vi "MotorControlMina4 with Joystick control2.vi"() -> ()   [LabVIEW 2014]
uses:
  <vilib>/Utility/inputDevices.llb/joystickAcquire.vi
  <vilib>/Utility/inputDevices.llb/closeJoystick.vi
panel:
  out "joystick info":T1(array[cluster])
  in  "Stop":bool
  out "InstrumentMode":T2(ring)=enum."Shutdown"
  in  "XMotorRef":refnum<k7>(container)
  in  "YMotorRef":refnum<k7>(container)
  in  "ZMotorRef":refnum<k7>(container)
  out "JoystOffset":T3={"XOffset"=-99999, "YOffset"=-99999, "ZOffset"=-99999}
  out "RelJoyPos":T4
  in  "InterfaceSelector":T5(tab)
  in  "GoToTopDisp":bool
  in  "GoToBottDisp":bool
  in  "GoToExpLoc":bool
  in  "SaveTopDisp":bool
  in  "SaveBottDisp":bool
  in  "SaveExpLoc":bool
  out "Top Dispenser":T6={"X Pos (mm)"=0.5532008, "Y Pos (mm)"=0.030929338, "Z Pos (mm)"=0.77973413} {"Y Pos (mm)" format="%.3f"; "Z Pos (mm)" format="%.3f"; "X Pos (mm)" format="%.3f"}
  out "Bottom Dispenser":T6={"X Pos (mm)"=0.600309, "Y Pos (mm)"=-1.1540928, "Z Pos (mm)"=0.7938141} {"Y Pos (mm)" format="%.3f"; "Z Pos (mm)" format="%.3f"; "X Pos (mm)" format="%.3f"}
  out "Experiment Region":T6={"X Pos (mm)"=1.4278219, "Y Pos (mm)"=-0.74810517, "Z Pos (mm)"=0.7938141} {"Y Pos (mm)" format="%.3f"; "Z Pos (mm)" format="%.3f"; "X Pos (mm)" format="%.3f"}
  in  "PreviewPanel":T7(tab)
  in  "Z Motor Settings":T8={"Joyst Min Signal"=10.0, "Joyst Max Signal"=30000.0, "Vmax (mm/s)"=0.005, "Acc (mm/s/s)"=0.2, "+ JoystDirection"=2, "- JoystDirection"=1} {"Acc (mm/s/s)" format="%#.3f"; "Vmax (mm/s)" format="%#.3f"}
  in  "Y Motor Settings":T8={"Joyst Min Signal"=10.0, "Joyst Max Signal"=20000.0, "Vmax (mm/s)"=0.03, "Acc (mm/s/s)"=0.5, "+ JoystDirection"=1, "- JoystDirection"=2} {"Acc (mm/s/s)" format="%#.3f"; "Vmax (mm/s)" format="%#.3f"}
  in  "X Motor Settings":T8={"Joyst Min Signal"=10.0, "Joyst Max Signal"=20000.0, "Vmax (mm/s)"=0.03, "Acc (mm/s/s)"=0.5, "+ JoystDirection"=2, "- JoystDirection"=1} {"Acc (mm/s/s)" format="%#.3f"; "Vmax (mm/s)" format="%#.3f"}
  in  "Motor Cruise Param":T9={"X Acc (mm/s^2)"=0.3, "X Vmax (mm/s)"=0.3, "Y Acc (mm/s^2)"=0.3, "Y Vmax (mm/s)"=0.3, "Z Acc (mm/s^2)"=0.1, "Z Vmax (mm/s)"=0.1}
  in  "Motor Limits":T10={"XMin"=-0.8, "XMax"=3.0, "YMin"=-2.0, "YMax"=2.0, "ZMin"=0.0, "ZMax"=2.0}
  in  "Steerable Mirror Calibration":T11={"Hor. Scaling (nm/V)"=760.0, "Vert. Scaling (nm/V)"=760.0, "Hor. Mirr. Offset (V)"=0.0, "Vert. Mirr. Offset (V)"=0.0}
  in  "Steerable \nTrap\n(F12)":bool
  in  "Fixed\nTrap\n(F11)":bool
  in  "Align Traps Vertically":bool
  in  "MaxHorizontalTrapSeparation":bool
  out "X Motor State":T12={"Direction"=0, "Vel (mm/s)"=0.0, "IsActive?"=FALSE, "Pos (mm)"=-0.2957381} {"Pos (mm)" format="%#.3f"; "Vel (mm/s)" format="%#.4f"}
  out "Y Motor State":T12={"Direction"=0, "Vel (mm/s)"=0.0, "IsActive?"=FALSE, "Pos (mm)"=0.016441232} {"Pos (mm)" format="%#.3f"; "Vel (mm/s)" format="%#.4f"}
  out "Z Motor State":T12={"Direction"=0, "Vel (mm/s)"=0.0, "IsActive?"=FALSE, "Pos (mm)"=-0.26253498} {"Pos (mm)" format="%#.3f"; "Vel (mm/s)" format="%#.4f"}
  out "Move Z":bool
  out "Move XY":bool
  in  "MotorLoopDelay":u32=100
  in  "StopPassiveMode":bool caption="stop"
  in  "PMVertSlider(V)":dbl(slide)=0.005145263671875 scale=0.0..10.0 scale format="%#_3f"
  in  "PMHorizSlider(V)":dbl(slide)=0.0045623779296875 scale=2.0..10.0
  out "IsPassiveModeActive?":bool caption="stop"
  out "Force TrapA":cluster{"x":dbl[], "y":dbl[]}[](graph)
  out "Noise-Ext":cluster{"x":dbl[], "y":dbl[]}[](graph)
  out "Force TrapB":cluster{"x":dbl[], "y":dbl[]}[](graph)
  out "IsOffsetModeActive?":bool caption="stop"
  in  "StopOffset":bool caption="stop"
  out "IsForceExtActive?":bool=TRUE
  in  "StopForceExtension":bool caption="stop"
  # "ClpXP Optical Tweezers"
  # "Chamber Locations"
  # "Need a Button Here that would read the \nNormalized Offset and save it"
  # "Off"
  # "On"
  # "Off"
  # "On"
  # "Thorlabs Motor Status"
  # "Passive Mode"
  # "when I switch tabs from the passive mode to basic mode, the recording doesn't stop"
  # "The sliders don't do anything in passive mode, fix it"
  # "Whenever I click on Ackquire Offset, it goes back to the basic operation, then I have to ckick again"
  # "Trap Motion Control"
  # "Steerable Mirror Info"
  # "Zero-Force Offset Mode"
  # "High Frequency Data Acquisition"
  # "Adjust the length of acquisition time"
  # "Force-Extension Mode"
  # "Y"
  # "+"
  # "X"
  # "-"
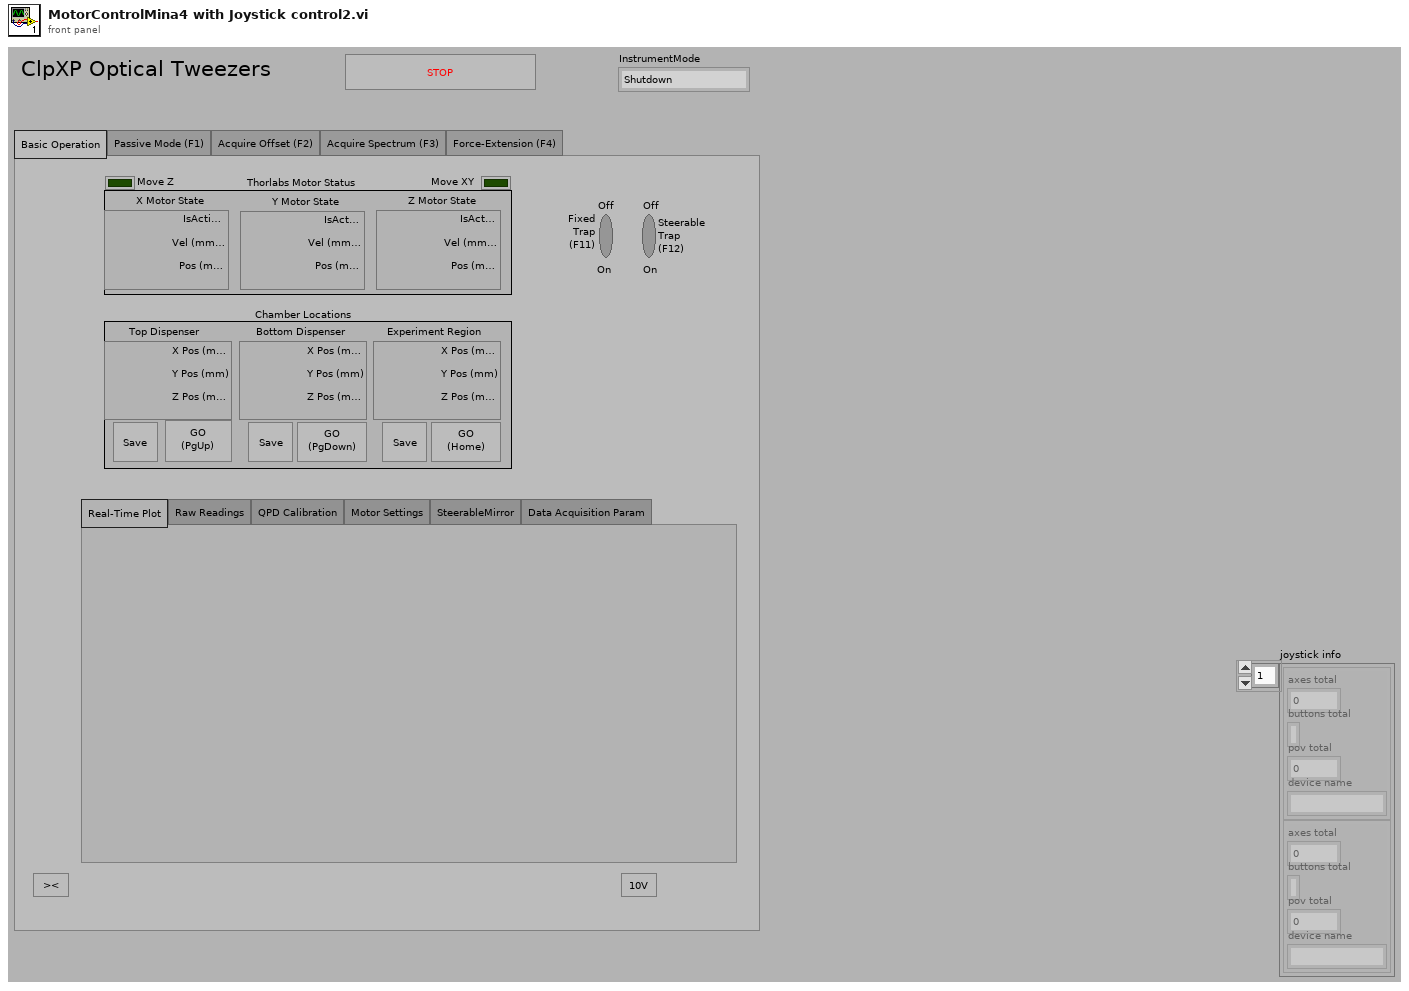
[diagram p1: front panel]
types:
  T1 = cluster{"axes total":u32, "buttons total":u32, "pov total":u32, "device name":string}[]
  T2 = enum16{"InitializeJoystick", "InitializeMotors", "BasicMode", "PassiveMode", "AcquireOffsetMode", "AcquireSpectrumMode", "Force-ExtensionMode", "Shutdown"}
  T3 = cluster{"XOffset":i32, "YOffset":i32, "ZOffset":i32}
  T4 = cluster{"XRelPos":i32, "YRelPos":i32, "ZRelPos":i32}
  T5 = enum32{"Basic Operation", "Passive Mode (F1)", "Acquire Offset (F2)", "Acquire Spectrum (F3)", "Force-Extension (F4)"}
  T6 = cluster{"X Pos (mm)":sgl, "Y Pos (mm)":sgl, "Z Pos (mm)":sgl}
  T7 = enum32{"Real-Time Plot", "Raw Readings", "QPD Calibration", "Motor Settings", "SteerableMirror", "Data Acquisition Param"}
  T8 = cluster{"Joyst Min Signal":dbl, "Joyst Max Signal":dbl, "Vmax (mm/s)":sgl, "Acc (mm/s/s)":sgl, "+ JoystDirection":i32, "- JoystDirection":i32}
  T9 = cluster{"X Acc (mm/s^2)":sgl, "X Vmax (mm/s)":sgl, "Y Acc (mm/s^2)":sgl, "Y Vmax (mm/s)":sgl, "Z Acc (mm/s^2)":sgl, "Z Vmax (mm/s)":sgl}
  T10 = cluster{"XMin":sgl, "XMax":sgl, "YMin":sgl, "YMax":sgl, "ZMin":sgl, "ZMax":sgl}
  T11 = cluster{"Hor. Scaling (nm/V)":dbl, "Vert. Scaling (nm/V)":dbl, "Hor. Mirr. Offset (V)":dbl, "Vert. Mirr. Offset (V)":dbl}
  T12 = cluster{"Direction":i32, "Vel (mm/s)":sgl, "IsActive?":bool, "Pos (mm)":sgl}
  T13 = cluster{"XMotorRef":refnum<k7>, "YMotorRef":refnum<k7>, "ZMotorRef":refnum<k7>}
  T14 = cluster{"Motor Reference":refnum<k7>, "Motor Reference":refnum<k7>, "Motor Reference":refnum<k7>}
  T15 = cluster{"X axis":i32, "Y axis":i32, "Z axis":i32, "X axis rotation":i32, "Y axis rotation":i32, "Z axis rotation":i32, "U axis":i32, "V axis":i32}
  T16 = cluster{"button 1":bool, "button 2":bool, "button 3":bool, "button 4":bool, "button 5":bool, "button 6":bool, "button 7":bool, "button 8":bool, "button 9":bool, "button 10":bool, "button 11":bool, "button 12":bool, "button 13":bool, "button 14":bool, "button 15":bool, "button 16":bool, "button 17":bool, "button 18":bool, "button 19":bool, "button 20":bool, "button 21":bool, "button 22":bool, "button 23":bool, "button 24":bool, "button 25":bool, "button 26":bool, "button 27":bool, "button 28":bool, "button 29":bool, "button 30":bool, "button 31":bool, "button 32":bool}
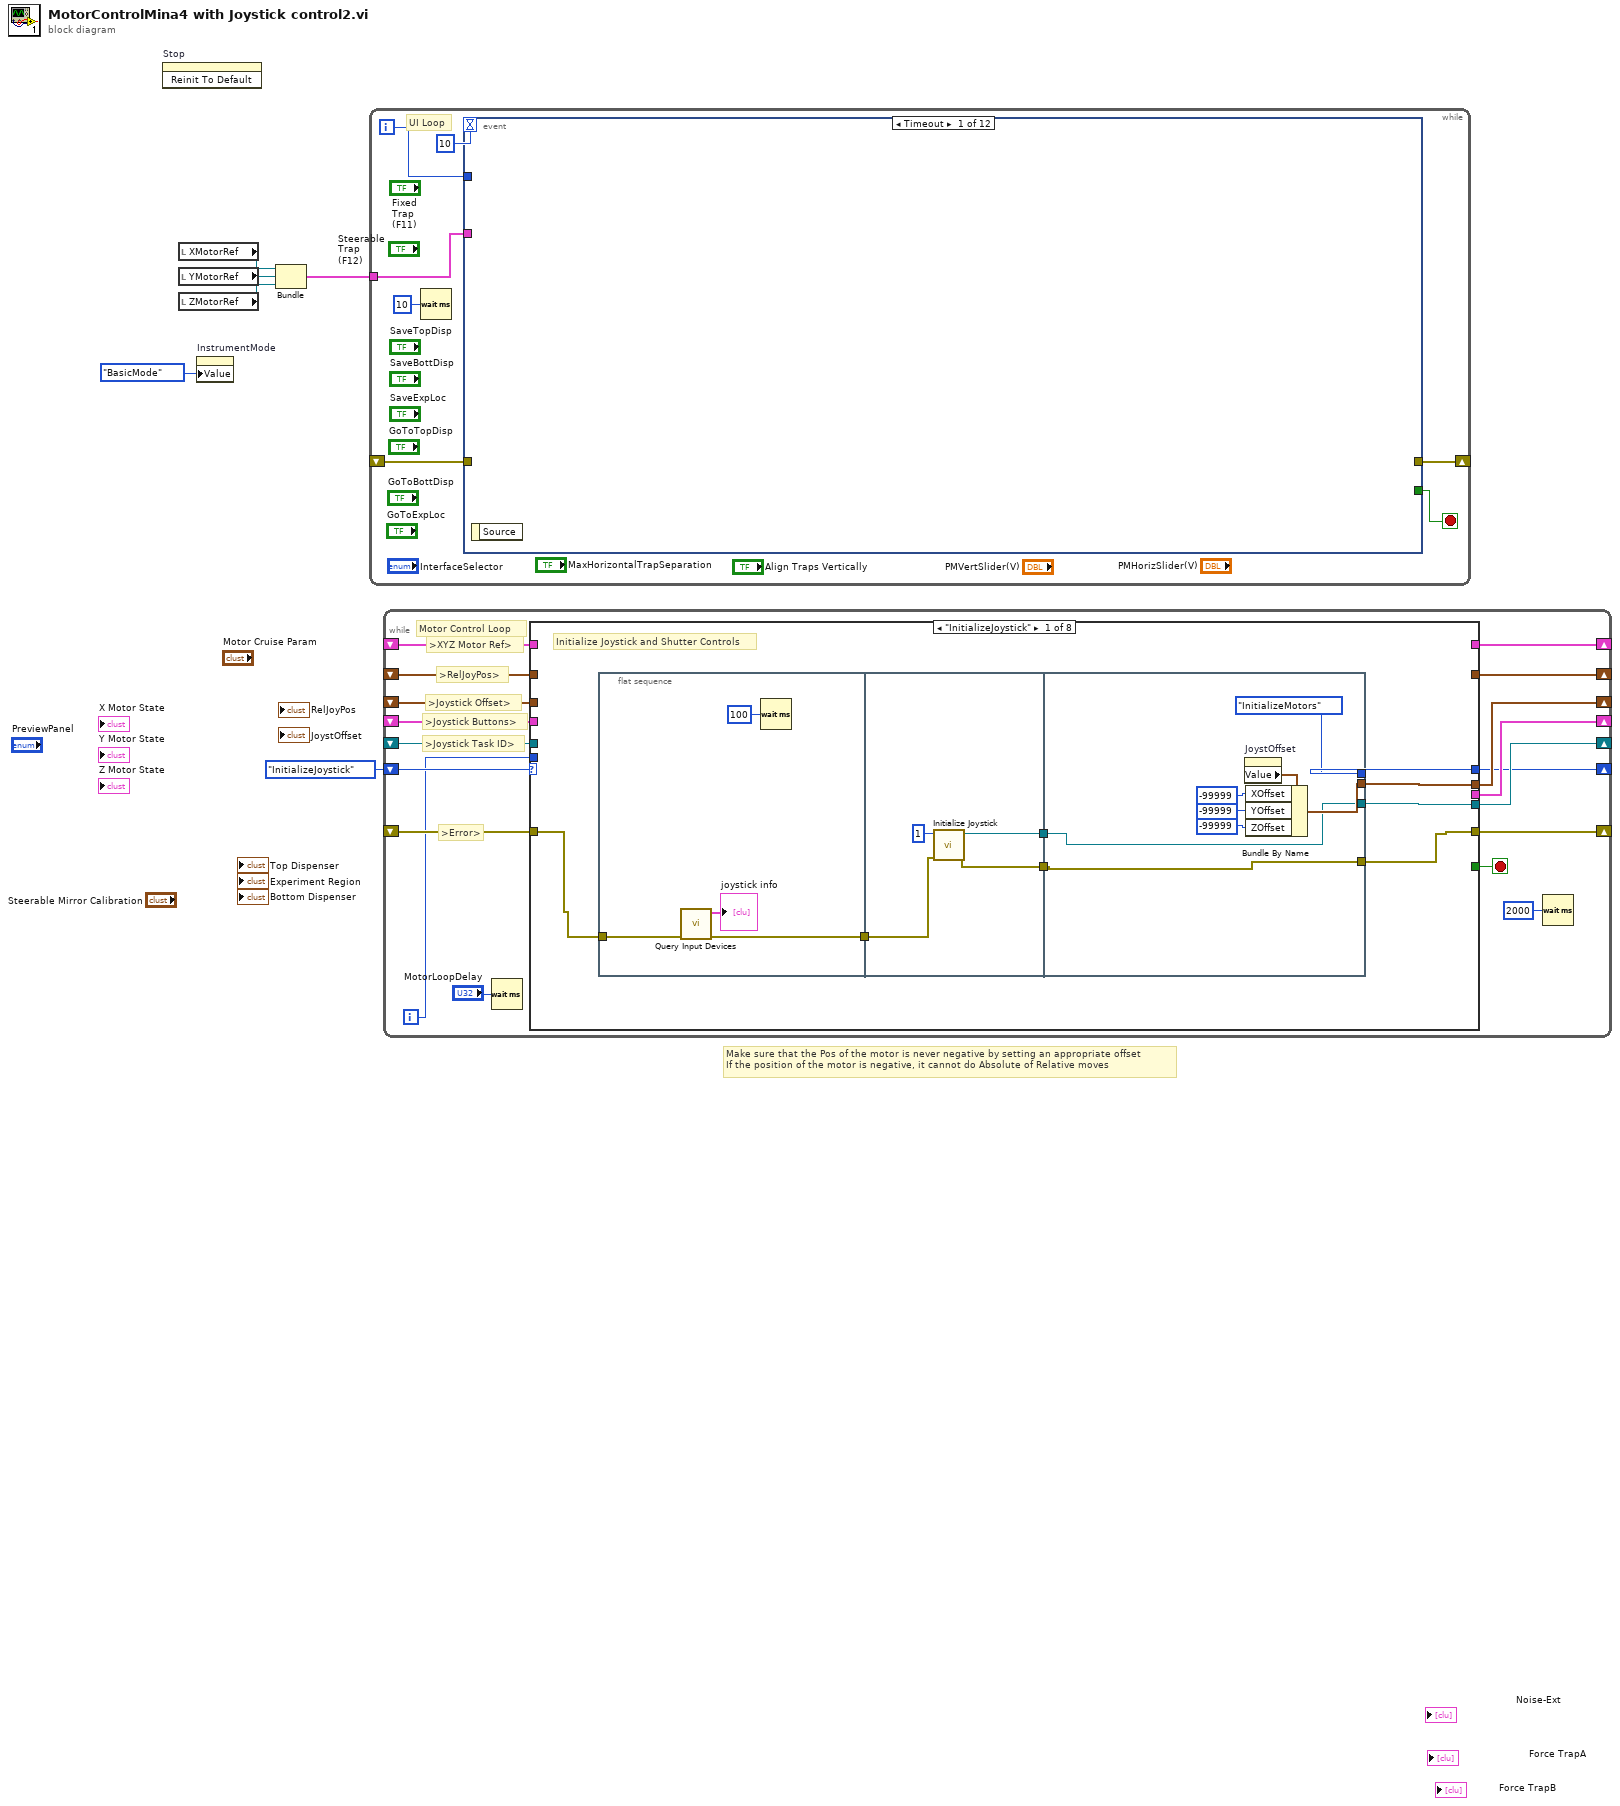
[diagram p0: block diagram]
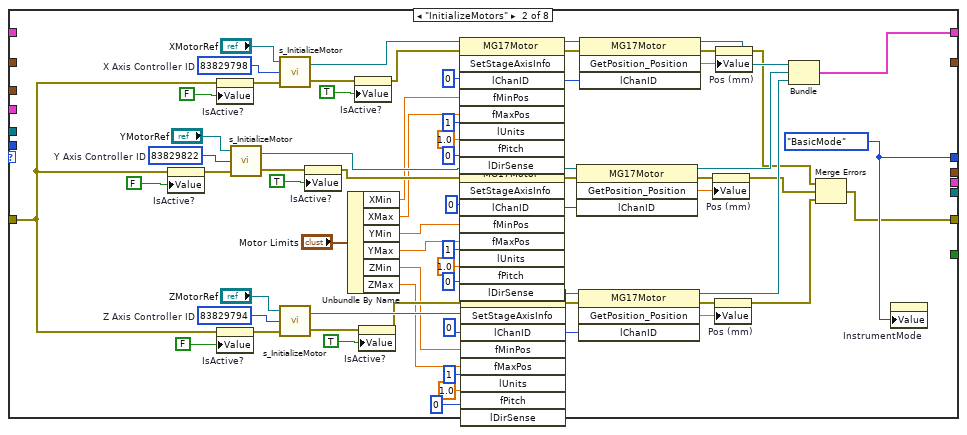
[diagram p2: hidden frame]
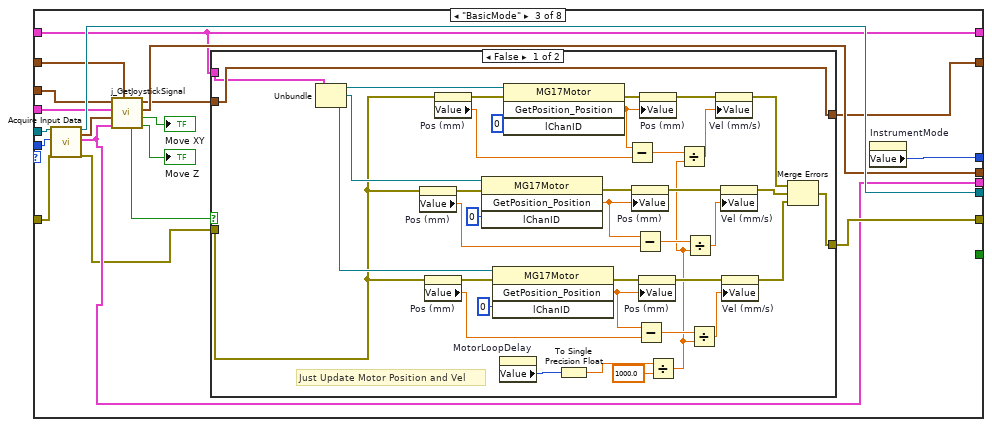
[diagram p3: hidden frame]
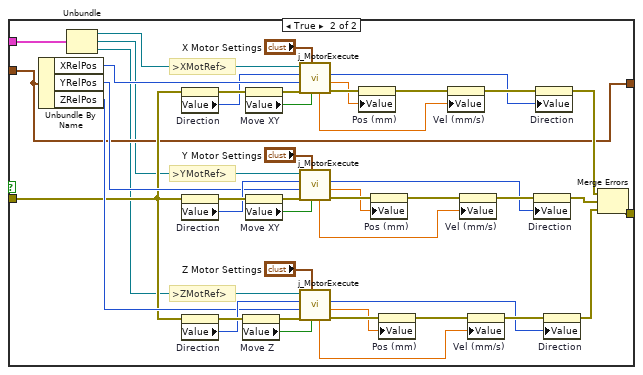
[diagram p4: hidden frame]
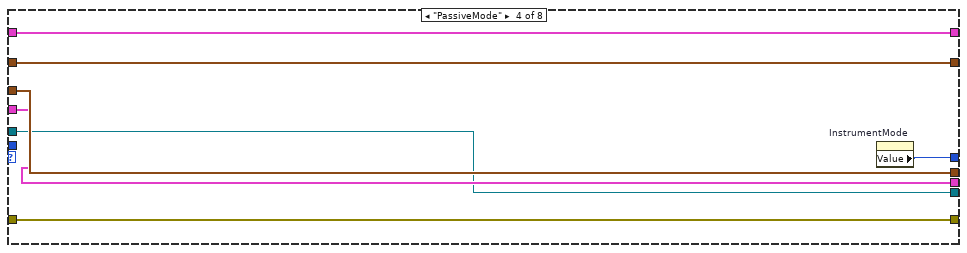
[diagram p5: hidden frame]
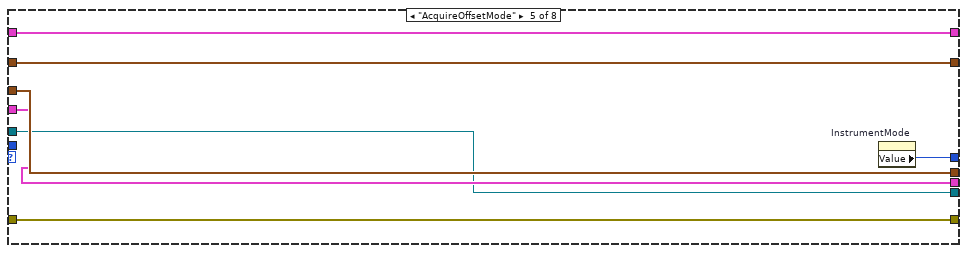
[diagram p6: hidden frame]
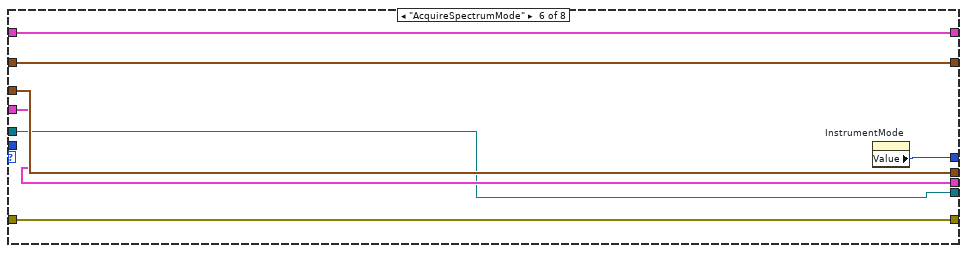
[diagram p7: hidden frame]
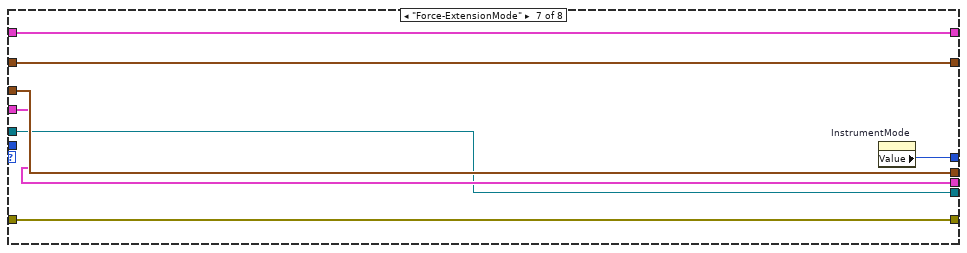
[diagram p8: hidden frame]
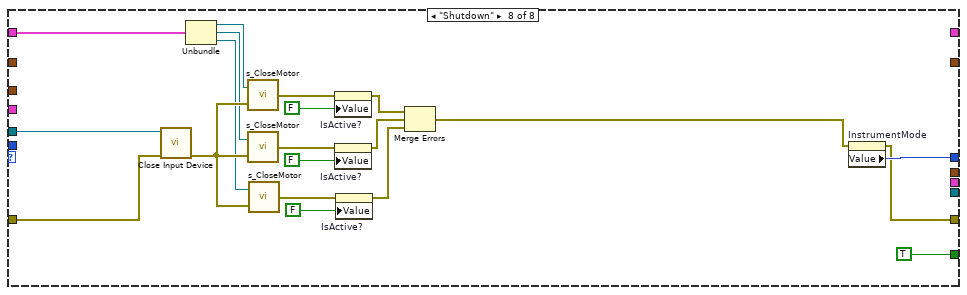
[diagram p9: hidden frame]
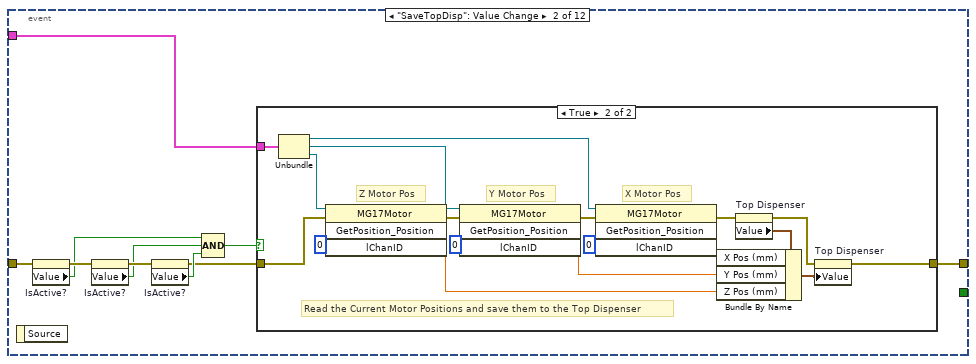
[diagram p10: hidden frame]
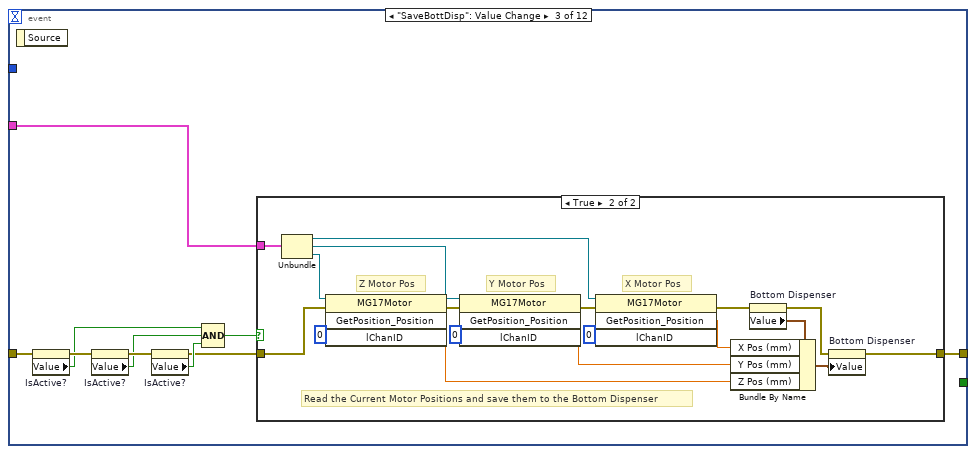
[diagram p12: hidden frame]
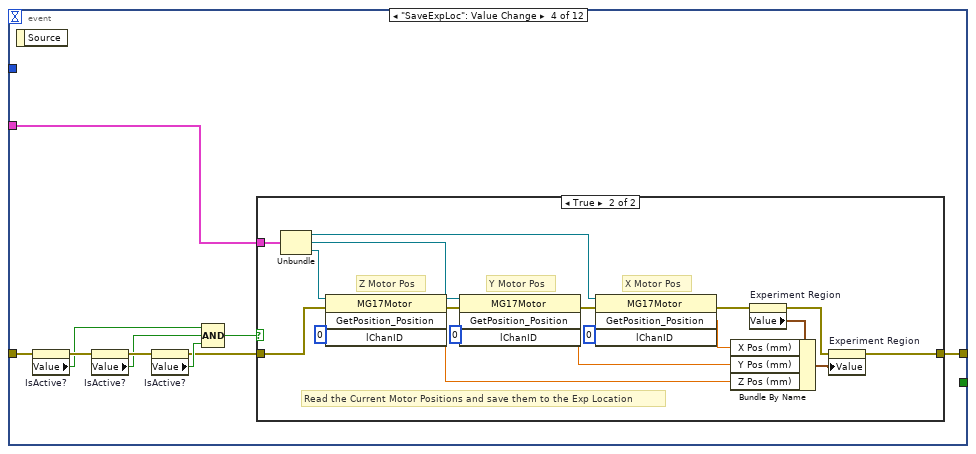
[diagram p14: hidden frame]
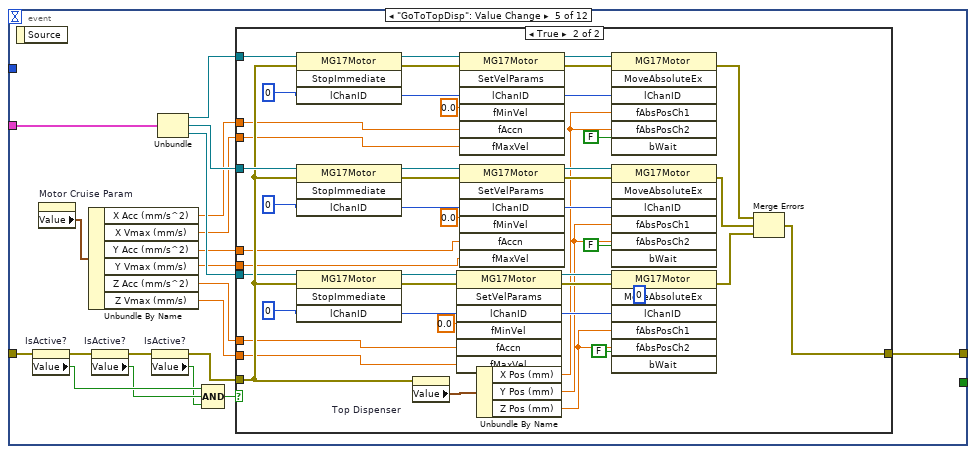
[diagram p16: hidden frame]
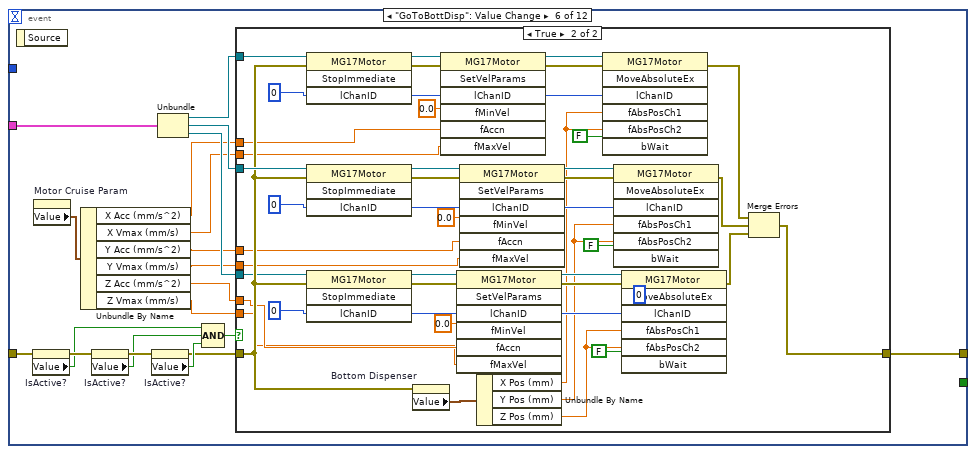
[diagram p18: hidden frame]
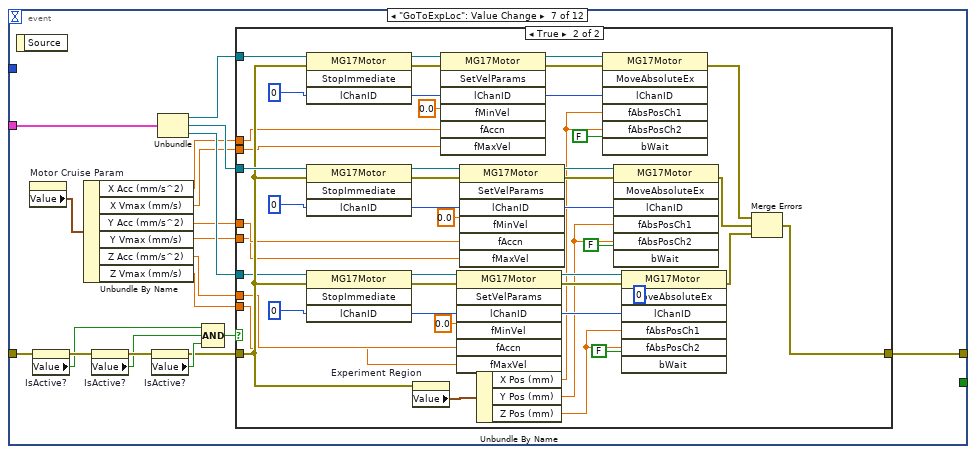
[diagram p20: hidden frame]
diagram:
  # "Make sure that the Pos of the motor is never negative by setting an appropriate offset\nIf the position of the motor is negative, it cannot do Absolute of Relative moves"
  n1 = invoke on="Stop" class="Bool" method="Reinit To Default"() -> ()  [unwired: 3 in, 3 out]
  n2 = local read "XMotorRef"() -> (w6:refnum<k7>)
  n3 = local read "YMotorRef"() -> (w5:refnum<k7>)
  n4 = local read "ZMotorRef"() -> (w4:refnum<k7>)
  n5 = property on="InstrumentMode" class="Enum (strict)"("Value"=T2."BasicMode") -> ()  [unwired: 2 in, 2 out]
  n6 = Bundle("XMotorRef"=w6, "YMotorRef"=w5, "ZMotorRef"=w4) -> (w3:T13)  [unwired: 1 in]
  n7 = while {
    shift-right: [w12] -> _
    shift-left: _ -> [w11]
    tunnel: w3 -> [w10]
    i -> [w8]
    stop <- w9 stop-if-true
    # "UI Loop"
    n8 = Wait (ms)(milliseconds to wait=u32 10) -> ()  [unwired: 1 out]
    n9 = event shown="[0] Timeout" {
      selector: _ -> [_ _ _ _ _ _ _ _ _ _ _ _]
      dyn-events: _ -> [_ _ _ _ _ _ _ _ _ _ _ _]
      timeout: 10 -> [_ _ _ _ _ _ _ _ _ _ _ _]
      tunnel: [_ w16 w45 w74 w113 w179 w245 w299 _ _ _ w327] -> w12
      tunnel: w11 -> [_ w15 w44 w73 w112 w178 w244 w299 _ _ _ w327]
      tunnel: [_ _ _ _ _ _ _ _ _ _ _ "Stop"] -> w9
      tunnel: w10 -> [_ w14 w43 w72 w111 w177 w243 _ _ _ _ _]
      tunnel: w8 -> [_ _ _ _ _ _ _ _ _ _ _ _]
      event Timeout {
        n10 = event-data() -> ()  [unwired: 1 in, 1 out]
      }
      event "SaveTopDisp": Value Change {
        n11 = event-data() -> ()  [unwired: 1 in, 1 out]
        n12 = property on="IsActive?" class="Bool (strict)"(error in=w15) -> (error out=w23:errorcluster, "Value"=w21:bool)  [unwired: 1 in, 1 out]
        n13 = property on="IsActive?" class="Bool (strict)"(error in=w23) -> (error out=w22:errorcluster, "Value"=w20:bool)  [unwired: 1 in, 1 out]
        n14 = property on="IsActive?" class="Bool (strict)"(error in=w22) -> (error out=w17:errorcluster, "Value"=w19:bool)  [unwired: 1 in, 1 out]
        n15 = Compound Arithmetic op=AND(w21, w20, w19) -> (w18:bool)
        n16 = case shown="True" w18 {
          tunnel: w17 -> [w24 w42]
          tunnel: [w24 w29] -> w16
          tunnel: w14 -> [_ w28]
          frame False {
          }
          frame True {
            # "Read the Current Motor Positions and save them to the Top Dispenser"
            # "X Motor Pos"
            # "Y Motor Pos"
            # "Z Motor Pos"
            n17 = Unbundle(w28) -> ("XMotorRef"=w25:refnum<k7>, "YMotorRef"=w26:refnum<k7>, "ZMotorRef"=w27:refnum<k7>)
            n18 = invoke class="MG17Motor" method="GetPosition_Position"(reference=w27, error in=w42, "lChanID"=0) -> (error out=w39:errorcluster, "GetPosition_Position"=w32:sgl)  [unwired: 1 in, 2 out]
            n19 = invoke class="MG17Motor" method="GetPosition_Position"(reference=w26, error in=w39, "lChanID"=0) -> (error out=w37:errorcluster, "GetPosition_Position"=w31:sgl)  [unwired: 1 in, 2 out]
            n20 = invoke class="MG17Motor" method="GetPosition_Position"(reference=w25, error in=w37, "lChanID"=0) -> (error out=w36:errorcluster, "GetPosition_Position"=w30:sgl)  [unwired: 1 in, 2 out]
            n21 = property on="Top Dispenser" class="Clust (strict)"(error in=w36) -> (error out=w35:errorcluster, "Value"=w34:T6)  [unwired: 1 in, 1 out]
            n22 = Bundle By Name(cluster=w34, "X Pos (mm)"=w30, "Y Pos (mm)"=w31, "Z Pos (mm)"=w32) -> (w33:T6)
            n23 = property on="Top Dispenser" class="Clust (strict)"(error in=w35, "Value"=w33) -> (error out=w29:errorcluster)  [unwired: 1 in, 1 out]
          }
        }
      }
      event "SaveBottDisp": Value Change {
        n24 = event-data() -> ()  [unwired: 1 in, 1 out]
        n25 = property on="IsActive?" class="Bool (strict)"(error in=w44) -> (error out=w52:errorcluster, "Value"=w50:bool)  [unwired: 1 in, 1 out]
        n26 = property on="IsActive?" class="Bool (strict)"(error in=w52) -> (error out=w51:errorcluster, "Value"=w49:bool)  [unwired: 1 in, 1 out]
        n27 = property on="IsActive?" class="Bool (strict)"(error in=w51) -> (error out=w46:errorcluster, "Value"=w48:bool)  [unwired: 1 in, 1 out]
        n28 = Compound Arithmetic op=AND(w50, w49, w48) -> (w47:bool)
        n29 = case shown="True" w47 {
          tunnel: w46 -> [w53 w71]
          tunnel: [w53 w58] -> w45
          tunnel: w43 -> [_ w57]
          frame False {
          }
          frame True {
            # "Read the Current Motor Positions and save them to the Bottom Dispenser"
            # "X Motor Pos"
            # "Y Motor Pos"
            # "Z Motor Pos"
            n30 = Unbundle(w57) -> ("XMotorRef"=w54:refnum<k7>, "YMotorRef"=w55:refnum<k7>, "ZMotorRef"=w56:refnum<k7>)
            n31 = invoke class="MG17Motor" method="GetPosition_Position"(reference=w56, error in=w71, "lChanID"=0) -> (error out=w68:errorcluster, "GetPosition_Position"=w61:sgl)  [unwired: 1 in, 2 out]
            n32 = invoke class="MG17Motor" method="GetPosition_Position"(reference=w55, error in=w68, "lChanID"=0) -> (error out=w66:errorcluster, "GetPosition_Position"=w60:sgl)  [unwired: 1 in, 2 out]
            n33 = invoke class="MG17Motor" method="GetPosition_Position"(reference=w54, error in=w66, "lChanID"=0) -> (error out=w65:errorcluster, "GetPosition_Position"=w59:sgl)  [unwired: 1 in, 2 out]
            n34 = property on="Bottom Dispenser" class="Clust (strict)"(error in=w65) -> (error out=w64:errorcluster, "Value"=w63:T6)  [unwired: 1 in, 1 out]
            n35 = Bundle By Name(cluster=w63, "X Pos (mm)"=w59, "Y Pos (mm)"=w60, "Z Pos (mm)"=w61) -> (w62:T6)
            n36 = property on="Bottom Dispenser" class="Clust (strict)"(error in=w64, "Value"=w62) -> (error out=w58:errorcluster)  [unwired: 1 in, 1 out]
          }
        }
      }
      event "SaveExpLoc": Value Change {
        n37 = event-data() -> ()  [unwired: 1 in, 1 out]
        n38 = property on="IsActive?" class="Bool (strict)"(error in=w73) -> (error out=w81:errorcluster, "Value"=w79:bool)  [unwired: 1 in, 1 out]
        n39 = property on="IsActive?" class="Bool (strict)"(error in=w81) -> (error out=w80:errorcluster, "Value"=w78:bool)  [unwired: 1 in, 1 out]
        n40 = property on="IsActive?" class="Bool (strict)"(error in=w80) -> (error out=w75:errorcluster, "Value"=w77:bool)  [unwired: 1 in, 1 out]
        n41 = Compound Arithmetic op=AND(w79, w78, w77) -> (w76:bool)
        n42 = case shown="True" w76 {
          tunnel: w75 -> [w82 w100]
          tunnel: [w82 w87] -> w74
          tunnel: w72 -> [_ w86]
          frame False {
          }
          frame True {
            # "Read the Current Motor Positions and save them to the Exp Location"
            # "X Motor Pos"
            # "Y Motor Pos"
            # "Z Motor Pos"
            n43 = Unbundle(w86) -> ("XMotorRef"=w83:refnum<k7>, "YMotorRef"=w84:refnum<k7>, "ZMotorRef"=w85:refnum<k7>)
            n44 = invoke class="MG17Motor" method="GetPosition_Position"(reference=w85, error in=w100, "lChanID"=0) -> (error out=w97:errorcluster, "GetPosition_Position"=w90:sgl)  [unwired: 1 in, 2 out]
            n45 = invoke class="MG17Motor" method="GetPosition_Position"(reference=w84, error in=w97, "lChanID"=0) -> (error out=w95:errorcluster, "GetPosition_Position"=w89:sgl)  [unwired: 1 in, 2 out]
            n46 = invoke class="MG17Motor" method="GetPosition_Position"(reference=w83, error in=w95, "lChanID"=0) -> (error out=w94:errorcluster, "GetPosition_Position"=w88:sgl)  [unwired: 1 in, 2 out]
            n47 = property on="Experiment Region" class="Clust (strict)"(error in=w94) -> (error out=w93:errorcluster, "Value"=w92:T6)  [unwired: 1 in, 1 out]
            n48 = Bundle By Name(cluster=w92, "X Pos (mm)"=w88, "Y Pos (mm)"=w89, "Z Pos (mm)"=w90) -> (w91:T6)
            n49 = property on="Experiment Region" class="Clust (strict)"(error in=w93, "Value"=w91) -> (error out=w87:errorcluster)  [unwired: 1 in, 1 out]
          }
        }
      }
      event "GoToTopDisp": Value Change {
        n50 = event-data() -> ()  [unwired: 1 in, 1 out]
        n51 = property on="IsActive?" class="Bool (strict)"(error in=w112) -> (error out=w120:errorcluster, "Value"=w118:bool)  [unwired: 1 in, 1 out]
        n52 = property on="Motor Cruise Param" class="Clust (strict)"() -> ("Value"=w101:T9)  [unwired: 2 in, 2 out]
        n53 = Unbundle By Name(w101) -> ("X Acc (mm/s^2)"=w105:sgl, "X Vmax (mm/s)"=w104:sgl, "Y Acc (mm/s^2)"=w103:sgl, "Y Vmax (mm/s)"=w102:sgl, "Z Acc (mm/s^2)"=w107:sgl, "Z Vmax (mm/s)"=w106:sgl)
        n54 = property on="IsActive?" class="Bool (strict)"(error in=w120) -> (error out=w119:errorcluster, "Value"=w117:bool)  [unwired: 1 in, 1 out]
        n55 = property on="IsActive?" class="Bool (strict)"(error in=w119) -> (error out=w114:errorcluster, "Value"=w116:bool)  [unwired: 1 in, 1 out]
        n56 = Unbundle(w111) -> ("XMotorRef"=w110:refnum<k7>, "YMotorRef"=w109:refnum<k7>, "ZMotorRef"=w108:refnum<k7>)
        n57 = Compound Arithmetic op=AND(w118, w117, w116) -> (w115:bool)
        n58 = case shown="True" w115 {
          tunnel: w114 -> [w121 w141]
          tunnel: [w121 w137] -> w113
          tunnel: w110 -> [_ w164]
          tunnel: w109 -> [_ w149]
          tunnel: w108 -> [_ w136]
          tunnel: w107 -> [_ w127]
          tunnel: w106 -> [_ w126]
          tunnel: w105 -> [_ w125]
          tunnel: w104 -> [_ w124]
          tunnel: w103 -> [_ w123]
          tunnel: w102 -> [_ w122]
          frame False {
          }
          frame True {
            (unwired) 0 ("lChanID")
            n59 = invoke class="MG17Motor" method="StopImmediate"(reference=w164, error in=w141, "lChanID"=0) -> (reference out=w162:refnum<k7>, error out=w163:errorcluster, "lChanID"=w132:i32)  [unwired: 1 in, 1 out]
            n60 = invoke class="MG17Motor" method="StopImmediate"(reference=w149, error in=w141, "lChanID"=0) -> (reference out=w156:refnum<k7>, error out=w157:errorcluster, "lChanID"=w133:i32)  [unwired: 1 in, 1 out]
            n61 = invoke class="MG17Motor" method="StopImmediate"(reference=w136, error in=w141, "lChanID"=0) -> (reference out=w146:refnum<k7>, error out=w147:errorcluster, "lChanID"=w134:i32)  [unwired: 1 in, 1 out]
            n62 = property on="Top Dispenser" class="Clust (strict)"(error in=w141) -> ("Value"=w166:T6)  [unwired: 1 in, 2 out]
            n63 = invoke class="MG17Motor" method="SetVelParams"(reference=w146, error in=w147, "lChanID"=w134, "fMinVel"=sgl 0.0, "fAccn"=w127, "fMaxVel"=w126) -> (reference out=w145:refnum<k7>, error out=w144:errorcluster, "lChanID"=w143:i32)  [unwired: 1 in, 4 out]
            n64 = invoke class="MG17Motor" method="SetVelParams"(reference=w162, error in=w163, "lChanID"=w132, "fMinVel"=sgl 0.0, "fAccn"=w125, "fMaxVel"=w124) -> (reference out=w161:refnum<k7>, error out=w160:errorcluster, "lChanID"=w159:i32)  [unwired: 1 in, 4 out]
            n65 = invoke class="MG17Motor" method="SetVelParams"(reference=w156, error in=w157, "lChanID"=w133, "fMinVel"=sgl 0.0, "fAccn"=w123, "fMaxVel"=w122) -> (reference out=w154:refnum<k7>, error out=w153:errorcluster, "lChanID"=w152:i32)  [unwired: 1 in, 4 out]
            n66 = Unbundle By Name(w166) -> ("X Pos (mm)"=w130:sgl, "Y Pos (mm)"=w129:sgl, "Z Pos (mm)"=w128:sgl)
            n67 = invoke class="MG17Motor" method="MoveAbsoluteEx"(reference=w161, error in=w160, "lChanID"=w159, "fAbsPosCh1"=w130, "fAbsPosCh2"=w130, "bWait"=FALSE) -> (error out=w140:errorcluster)  [unwired: 1 in, 6 out]
            n68 = invoke class="MG17Motor" method="MoveAbsoluteEx"(reference=w154, error in=w153, "lChanID"=w152, "fAbsPosCh1"=w129, "fAbsPosCh2"=w129, "bWait"=FALSE) -> (error out=w139:errorcluster)  [unwired: 1 in, 6 out]
            n69 = invoke class="MG17Motor" method="MoveAbsoluteEx"(reference=w145, error in=w144, "lChanID"=w143, "fAbsPosCh1"=w128, "fAbsPosCh2"=w128, "bWait"=FALSE) -> (error out=w138:errorcluster)  [unwired: 1 in, 6 out]
            n70 = Merge Errors(w140, w139, w138) -> (w137:errorcluster)
          }
        }
      }
      event "GoToBottDisp": Value Change {
        n71 = event-data() -> ()  [unwired: 1 in, 1 out]
        n72 = property on="IsActive?" class="Bool (strict)"(error in=w178) -> (error out=w186:errorcluster, "Value"=w184:bool)  [unwired: 1 in, 1 out]
        n73 = property on="Motor Cruise Param" class="Clust (strict)"() -> ("Value"=w173:T9)  [unwired: 2 in, 2 out]
        n74 = Unbundle By Name(w173) -> ("X Acc (mm/s^2)"=w172:sgl, "X Vmax (mm/s)"=w171:sgl, "Y Acc (mm/s^2)"=w170:sgl, "Y Vmax (mm/s)"=w169:sgl, "Z Acc (mm/s^2)"=w168:sgl, "Z Vmax (mm/s)"=w167:sgl)
        n75 = property on="IsActive?" class="Bool (strict)"(error in=w186) -> (error out=w185:errorcluster, "Value"=w183:bool)  [unwired: 1 in, 1 out]
        n76 = property on="IsActive?" class="Bool (strict)"(error in=w185) -> (error out=w180:errorcluster, "Value"=w182:bool)  [unwired: 1 in, 1 out]
        n77 = Unbundle(w177) -> ("XMotorRef"=w176:refnum<k7>, "YMotorRef"=w175:refnum<k7>, "ZMotorRef"=w174:refnum<k7>)
        n78 = Compound Arithmetic op=AND(w184, w183, w182) -> (w181:bool)
        n79 = case shown="True" w181 {
          tunnel: w180 -> [w187 w207]
          tunnel: [w187 w203] -> w179
          tunnel: w176 -> [_ w230]
          tunnel: w175 -> [_ w215]
          tunnel: w174 -> [_ w202]
          tunnel: w172 -> [_ w193]
          tunnel: w171 -> [_ w192]
          tunnel: w170 -> [_ w191]
          tunnel: w169 -> [_ w190]
          tunnel: w168 -> [_ w189]
          tunnel: w167 -> [_ w188]
          frame False {
          }
          frame True {
            (unwired) 0 ("lChanID")
            n80 = invoke class="MG17Motor" method="StopImmediate"(reference=w230, error in=w207, "lChanID"=0) -> (reference out=w228:refnum<k7>, error out=w229:errorcluster, "lChanID"=w198:i32)  [unwired: 1 in, 1 out]
            n81 = invoke class="MG17Motor" method="StopImmediate"(reference=w215, error in=w207, "lChanID"=0) -> (reference out=w222:refnum<k7>, error out=w223:errorcluster, "lChanID"=w199:i32)  [unwired: 1 in, 1 out]
            n82 = invoke class="MG17Motor" method="StopImmediate"(reference=w202, error in=w207, "lChanID"=0) -> (reference out=w212:refnum<k7>, error out=w213:errorcluster, "lChanID"=w200:i32)  [unwired: 1 in, 1 out]
            n83 = property on="Bottom Dispenser" class="Clust (strict)"(error in=w207) -> ("Value"=w232:T6)  [unwired: 1 in, 2 out]
            n84 = invoke class="MG17Motor" method="SetVelParams"(reference=w228, error in=w229, "lChanID"=w198, "fMinVel"=sgl 0.0, "fAccn"=w193, "fMaxVel"=w192) -> (reference out=w227:refnum<k7>, error out=w226:errorcluster, "lChanID"=w225:i32)  [unwired: 1 in, 4 out]
            n85 = invoke class="MG17Motor" method="SetVelParams"(reference=w212, error in=w213, "lChanID"=w200, "fMinVel"=sgl 0.0, "fAccn"=w189, "fMaxVel"=w188) -> (reference out=w211:refnum<k7>, error out=w210:errorcluster, "lChanID"=w209:i32)  [unwired: 1 in, 4 out]
            n86 = invoke class="MG17Motor" method="SetVelParams"(reference=w222, error in=w223, "lChanID"=w199, "fMinVel"=sgl 0.0, "fAccn"=w191, "fMaxVel"=w190) -> (reference out=w220:refnum<k7>, error out=w219:errorcluster, "lChanID"=w218:i32)  [unwired: 1 in, 4 out]
            n87 = Unbundle By Name(w232) -> ("X Pos (mm)"=w196:sgl, "Y Pos (mm)"=w195:sgl, "Z Pos (mm)"=w194:sgl)
            n88 = invoke class="MG17Motor" method="MoveAbsoluteEx"(reference=w227, error in=w226, "lChanID"=w225, "fAbsPosCh1"=w196, "fAbsPosCh2"=w196, "bWait"=FALSE) -> (error out=w206:errorcluster)  [unwired: 1 in, 6 out]
            n89 = invoke class="MG17Motor" method="MoveAbsoluteEx"(reference=w220, error in=w219, "lChanID"=w218, "fAbsPosCh1"=w195, "fAbsPosCh2"=w195, "bWait"=FALSE) -> (error out=w205:errorcluster)  [unwired: 1 in, 6 out]
            n90 = invoke class="MG17Motor" method="MoveAbsoluteEx"(reference=w211, error in=w210, "lChanID"=w209, "fAbsPosCh1"=w194, "fAbsPosCh2"=w194, "bWait"=FALSE) -> (error out=w204:errorcluster)  [unwired: 1 in, 6 out]
            n91 = Merge Errors(w206, w205, w204) -> (w203:errorcluster)
          }
        }
      }
      event "GoToExpLoc": Value Change {
        n92 = event-data() -> ()  [unwired: 1 in, 1 out]
        n93 = property on="Motor Cruise Param" class="Clust (strict)"() -> ("Value"=w239:T9)  [unwired: 2 in, 2 out]
        n94 = property on="IsActive?" class="Bool (strict)"(error in=w244) -> (error out=w252:errorcluster, "Value"=w250:bool)  [unwired: 1 in, 1 out]
        n95 = Unbundle By Name(w239) -> ("X Acc (mm/s^2)"=w238:sgl, "X Vmax (mm/s)"=w237:sgl, "Y Acc (mm/s^2)"=w236:sgl, "Y Vmax (mm/s)"=w235:sgl, "Z Acc (mm/s^2)"=w234:sgl, "Z Vmax (mm/s)"=w233:sgl)
        n96 = property on="IsActive?" class="Bool (strict)"(error in=w252) -> (error out=w251:errorcluster, "Value"=w249:bool)  [unwired: 1 in, 1 out]
        n97 = property on="IsActive?" class="Bool (strict)"(error in=w251) -> (error out=w246:errorcluster, "Value"=w248:bool)  [unwired: 1 in, 1 out]
        n98 = Unbundle(w243) -> ("XMotorRef"=w242:refnum<k7>, "YMotorRef"=w241:refnum<k7>, "ZMotorRef"=w240:refnum<k7>)
        n99 = Compound Arithmetic op=AND(w250, w249, w248) -> (w247:bool)
        n100 = case shown="True" w247 {
          tunnel: w246 -> [w253 w273]
          tunnel: [w253 w269] -> w245
          tunnel: w242 -> [_ w296]
          tunnel: w241 -> [_ w281]
          tunnel: w240 -> [_ w268]
          tunnel: w238 -> [_ w259]
          tunnel: w237 -> [_ w258]
          tunnel: w236 -> [_ w257]
          tunnel: w235 -> [_ w256]
          tunnel: w234 -> [_ w255]
          tunnel: w233 -> [_ w254]
          frame False {
          }
          frame True {
            (unwired) 0 ("lChanID")
            n101 = invoke class="MG17Motor" method="StopImmediate"(reference=w296, error in=w273, "lChanID"=0) -> (reference out=w294:refnum<k7>, error out=w295:errorcluster, "lChanID"=w264:i32)  [unwired: 1 in, 1 out]
            n102 = invoke class="MG17Motor" method="StopImmediate"(reference=w281, error in=w273, "lChanID"=0) -> (reference out=w288:refnum<k7>, error out=w289:errorcluster, "lChanID"=w265:i32)  [unwired: 1 in, 1 out]
            n103 = invoke class="MG17Motor" method="StopImmediate"(reference=w268, error in=w273, "lChanID"=0) -> (reference out=w278:refnum<k7>, error out=w279:errorcluster, "lChanID"=w266:i32)  [unwired: 1 in, 1 out]
            n104 = property on="Experiment Region" class="Clust (strict)"(error in=w273) -> ("Value"=w298:T6)  [unwired: 1 in, 2 out]
            n105 = invoke class="MG17Motor" method="SetVelParams"(reference=w294, error in=w295, "lChanID"=w264, "fMinVel"=sgl 0.0, "fAccn"=w259, "fMaxVel"=w258) -> (reference out=w293:refnum<k7>, error out=w292:errorcluster, "lChanID"=w291:i32)  [unwired: 1 in, 4 out]
            n106 = invoke class="MG17Motor" method="SetVelParams"(reference=w278, error in=w279, "lChanID"=w266, "fMinVel"=sgl 0.0, "fAccn"=w255, "fMaxVel"=w254) -> (reference out=w277:refnum<k7>, error out=w276:errorcluster, "lChanID"=w275:i32)  [unwired: 1 in, 4 out]
            n107 = invoke class="MG17Motor" method="SetVelParams"(reference=w288, error in=w289, "lChanID"=w265, "fMinVel"=sgl 0.0, "fAccn"=w257, "fMaxVel"=w256) -> (reference out=w286:refnum<k7>, error out=w285:errorcluster, "lChanID"=w284:i32)  [unwired: 1 in, 4 out]
            n108 = Unbundle By Name(w298) -> ("X Pos (mm)"=w262:sgl, "Y Pos (mm)"=w261:sgl, "Z Pos (mm)"=w260:sgl)
            n109 = invoke class="MG17Motor" method="MoveAbsoluteEx"(reference=w293, error in=w292, "lChanID"=w291, "fAbsPosCh1"=w262, "fAbsPosCh2"=w262, "bWait"=FALSE) -> (error out=w272:errorcluster)  [unwired: 1 in, 6 out]
            n110 = invoke class="MG17Motor" method="MoveAbsoluteEx"(reference=w286, error in=w285, "lChanID"=w284, "fAbsPosCh1"=w261, "fAbsPosCh2"=w261, "bWait"=FALSE) -> (error out=w271:errorcluster)  [unwired: 1 in, 6 out]
            n111 = invoke class="MG17Motor" method="MoveAbsoluteEx"(reference=w277, error in=w276, "lChanID"=w275, "fAbsPosCh1"=w260, "fAbsPosCh2"=w260, "bWait"=FALSE) -> (error out=w270:errorcluster)  [unwired: 1 in, 6 out]
            n112 = Merge Errors(w272, w271, w270) -> (w269:errorcluster)
          }
        }
      }
      event "InterfaceSelector": Value Change {
        n113 = event-data() -> ("NewVal"=w301:T5)  [unwired: 1 in]
        n114 = case shown="\"Force-Extension (F4)\"" w301 {
          tunnel: [T2."BasicMode" T2."PassiveMode" T2."AcquireOffsetMode" T2."AcquireSpectrumMode" T2."Force-ExtensionMode"] -> w300
          frame "Basic Operation" {
          }
          frame "Passive Mode (F1)" {
            n115 = property on="IsPassiveModeActive?" class="Bool (strict)"("Value"=TRUE ("StopOffset")) -> ()  [unwired: 2 in, 2 out]
          }
          frame "Acquire Offset (F2)" {
            n116 = property on="IsOffsetModeActive?" class="Bool (strict)"("Value"=TRUE ("StopOffset")) -> ()  [unwired: 2 in, 2 out]
          }
          frame "Acquire Spectrum (F3)" {
          }
          frame "Force-Extension (F4)" {
            n117 = property on="IsForceExtActive?" class="Bool (strict)"("Value"=TRUE ("StopOffset")) -> ()  [unwired: 2 in, 2 out]
          }
        }
        "InstrumentMode" <- w300
      }
      event "StopOffset": Value Change {
        n118 = event-data() -> ("NewVal"=w310:bool)  [unwired: 1 in, 5 out]
        n119 = case shown="True" w310 {
          frame False {
          }
          frame True {
            n120 = flat-sequence {
              frame #0 {
                n121 = Not(x="StopOffset") -> (.not. x?=→"IsOffsetModeActive?":bool)
              }
              frame #1 {
                n122 = property on="InterfaceSelector" class="TabCtl (strict)"("Value"=T5."Basic Operation" ("InterfaceSelector")) -> ()  [unwired: 2 in, 2 out]
                n123 = property on="InstrumentMode" class="Enum (strict)"("Value"=T2."BasicMode" ("InstrumentMode")) -> ()  [unwired: 2 in, 2 out]
              }
            }
          }
        }
      }
      event "StopPassiveMode": Value Change {
        n124 = event-data() -> ("NewVal"=w315:bool)  [unwired: 1 in, 5 out]
        n125 = case shown="True" w315 {
          frame False {
          }
          frame True {
            n126 = flat-sequence {
              frame #0 {
                n127 = Not(x="StopPassiveMode") -> (.not. x?=→"IsPassiveModeActive?":bool)
              }
              frame #1 {
                n128 = property on="InterfaceSelector" class="TabCtl (strict)"("Value"=T5."Basic Operation" ("InterfaceSelector")) -> ()  [unwired: 2 in, 2 out]
                n129 = property on="InstrumentMode" class="Enum (strict)"("Value"=T2."BasicMode" ("InstrumentMode")) -> ()  [unwired: 2 in, 2 out]
              }
            }
          }
        }
      }
      event "StopForceExtension": Value Change {
        n130 = event-data() -> ("NewVal"=w320:bool)  [unwired: 1 in, 5 out]
        n131 = case shown="True" w320 {
          frame False {
          }
          frame True {
            n132 = flat-sequence {
              frame #0 {
                n133 = Not(x="StopForceExtension") -> (.not. x?=→"IsForceExtActive?":bool)
              }
              frame #1 {
                n134 = property on="InterfaceSelector" class="TabCtl (strict)"("Value"=T5."Basic Operation" ("InterfaceSelector")) -> ()  [unwired: 2 in, 2 out]
                n135 = property on="InstrumentMode" class="Enum (strict)"("Value"=T2."BasicMode" ("InstrumentMode")) -> ()  [unwired: 2 in, 2 out]
              }
            }
          }
        }
      }
      event "Stop": Value Change {
        n136 = event-data() -> ()  [unwired: 1 in, 1 out]
        n137 = property on="InstrumentMode" class="Enum (strict)"("Value"=T2."Shutdown") -> ()  [unwired: 2 in, 2 out]
      }
    }
  }
  n138 = while {
    shift-right: [w331] -> _
    shift-left: T2."InitializeJoystick" -> [w330]
    shift-right: [w345] -> _
    shift-left: _ -> [w338]
    shift-right: [w342] -> _
    shift-left: _ -> [w344]
    shift-right: [w343] -> _
    shift-left: _ -> [w341]
    shift-right: [w340] -> _
    shift-left: _ -> [w339]
    shift-right: [w337] -> _
    shift-left: _ -> [w334]
    shift-right: [w335] -> _
    shift-left: _ -> [w336]
    i -> [w329]
    stop <- w332 stop-if-true
    # "Motor Control Loop"
    # ">Joystick Offset>"
    # ">RelJoyPos>"
    # ">XYZ Motor Ref>"
    # ">Error>"
    # ">Joystick Task ID>"
    # ">Joystick Buttons>"
    n139 = Wait (ms)(milliseconds to wait="MotorLoopDelay") -> ()  [unwired: 1 out]
    n140 = case shown="\"InitializeJoystick\"" w330 {
      tunnel: [w353 _ w453 w543 w550 w557 w564 _] -> w345
      tunnel: [w351 w371 w442 w547 w554 w561 w568 w587] -> w331
      tunnel: w344 -> [w350 w419 w455 w546 w553 w560 w567 w572]
      tunnel: [w352 _ w454 w541 w548 w555 w562 _] -> w343
      tunnel: [w349 w370 w446 w546 w553 w560 w567 w569] -> w342
      tunnel: w341 -> [_ _ w456 w541 w548 w555 w562 w571]
      tunnel: [_ _ w441 w542 w549 w556 w563 _] -> w340
      tunnel: w339 -> [_ _ w440 w542 w549 w556 w563 _]
      tunnel: w338 -> [_ _ w451 w543 w550 w557 w564 _]
      tunnel: [_ _ _ _ _ _ _ TRUE ("status")] -> w332
      tunnel: [_ w418 w445 w545 w552 w559 w566 _] -> w337
      tunnel: w334 -> [_ _ w445 w545 w552 w559 w566 w573]
      tunnel: [_ _ w443 w544 w551 w558 w565 _] -> w335
      tunnel: w336 -> [_ _ w452 w544 w551 w558 w565 _]
      tunnel: w329 -> [_ _ w438 _ _ _ _ _]
      frame "InitializeJoystick" {
        # "Initialize Joystick and Shutter Controls"
        n141 = flat-sequence {
          tunnel: w350 -> [w355]
          tunnel: [w354] -> w348
          tunnel: w348 -> [w360]
          tunnel: [w359] -> w347
          tunnel: [w358] -> w346
          tunnel: [w366] -> w353
          tunnel: [w362] -> w352
          tunnel: [T2."InitializeMotors"] -> w351
          tunnel: w347 -> [w363]
          tunnel: [w363] -> w349
          tunnel: w346 -> [w362]
          frame #0 {
            n142 = call <vilib>:"Query Input Devices.vi"("error in (no error)"=w355) -> ("error out"=w354:errorcluster, "joystick info"=→"joystick info":T1)  [unwired: 7 in, 2 out]
            n143 = Wait (ms)(milliseconds to wait=u32 100) -> ()  [unwired: 1 out]
          }
          frame #1 {
            n144 = call <vilib>:"Initialize Joystick.vi"("error in (no error)"=w360, "device index"=1) -> ("error out"=w359:errorcluster, "device ID"=w358:refnum<k1>)  [unwired: 8 in]
          }
          frame #2 {
            n145 = property on="JoystOffset" class="Clust (strict)"() -> ("Value"=w365:T3)  [unwired: 2 in, 2 out]
            n146 = Bundle By Name(cluster=w365, "XOffset"=-99999, "YOffset"=-99999, "ZOffset"=-99999) -> (w366:T3)
          }
        }
      }
      frame "InitializeMotors" {
        w371 = T2."BasicMode"
        w423 = 83829794  # Z Axis Controller ID
        w429 = 83829822  # Y Axis Controller ID
        w435 = 83829798  # X Axis Controller ID
        n147 = property on="IsActive?" class="Bool (strict)"(error in=w419, "Value"=FALSE ("IsYMotorActive?")) -> (error out=w430:errorcluster)  [unwired: 1 in, 1 out]
        n148 = property on="IsActive?" class="Bool (strict)"(error in=w419, "Value"=FALSE ("IsYMotorActive?")) -> (error out=w436:errorcluster)  [unwired: 1 in, 1 out]
        n149 = property on="IsActive?" class="Bool (strict)"(error in=w419, "Value"=FALSE ("IsYMotorActive?")) -> (error out=w424:errorcluster)  [unwired: 1 in, 1 out]
        n150 = call "s_InitializeMotor.vi"("Error In"=w430, "Servo Controller  ID"=w429, "Motor Reference In"="YMotorRef") -> ("Error Out"=w431:errorcluster, "Motor Reference"=w413:refnum<k7>)
        n151 = call "s_InitializeMotor.vi"("Error In"=w436, "Servo Controller  ID"=w435, "Motor Reference In"="XMotorRef") -> ("Error Out"=w437:errorcluster, "Motor Reference"=w417:refnum<k7>)
        n152 = call "s_InitializeMotor.vi"("Error In"=w424, "Servo Controller  ID"=w423, "Motor Reference In"="ZMotorRef") -> ("Error Out"=w425:errorcluster, "Motor Reference"=w410:refnum<k7>)
        n153 = property on="IsActive?" class="Bool (strict)"(error in=w431, "Value"=TRUE ("IsYMotorActive?")) -> (error out=w412:errorcluster)  [unwired: 1 in, 1 out]
        n154 = Unbundle By Name("Motor Limits") -> ("XMin"=w377:sgl, "XMax"=w376:sgl, "YMin"=w375:sgl, "YMax"=w374:sgl, "ZMin"=w373:sgl, "ZMax"=w372:sgl)
        n155 = property on="IsActive?" class="Bool (strict)"(error in=w437, "Value"=TRUE ("IsYMotorActive?")) -> (error out=w415:errorcluster)  [unwired: 1 in, 1 out]
        n156 = property on="IsActive?" class="Bool (strict)"(error in=w425, "Value"=TRUE ("IsYMotorActive?")) -> (error out=w409:errorcluster)  [unwired: 1 in, 1 out]
        n157 = invoke class="MG17Motor" method="SetStageAxisInfo"(reference=w417, error in=w415, "lChanID"=0, "fMinPos"=w377, "fMaxPos"=w376, "lUnits"=1, "fPitch"=sgl 1.0, "lDirSense"=0) -> (reference out=w408:refnum<k7>, error out=w407:errorcluster, "lChanID"=w406:i32)  [unwired: 1 in, 6 out]
        n158 = invoke class="MG17Motor" method="SetStageAxisInfo"(reference=w413, error in=w412, "lChanID"=0, "fMinPos"=w375, "fMaxPos"=w374, "lUnits"=1, "fPitch"=sgl 1.0, "lDirSense"=0) -> (reference out=w400:refnum<k7>, error out=w399:errorcluster, "lChanID"=w398:i32)  [unwired: 1 in, 6 out]
        n159 = invoke class="MG17Motor" method="SetStageAxisInfo"(reference=w410, error in=w409, "lChanID"=0, "fMinPos"=w373, "fMaxPos"=w372, "lUnits"=1, "fPitch"=sgl 1.0, "lDirSense"=0) -> (reference out=w395:refnum<k7>, error out=w394:errorcluster, "lChanID"=w393:i32)  [unwired: 1 in, 6 out]
        n160 = invoke class="MG17Motor" method="GetPosition_Position"(reference=w400, error in=w399, "lChanID"=w398) -> (reference out=w392:refnum<k7>, error out=w402:errorcluster, "GetPosition_Position"=w401:sgl)  [unwired: 1 in, 1 out]
        n161 = invoke class="MG17Motor" method="GetPosition_Position"(reference=w395, error in=w394, "lChanID"=w393) -> (reference out=w391:refnum<k7>, error out=w397:errorcluster, "GetPosition_Position"=w396:sgl)  [unwired: 1 in, 1 out]
        n162 = invoke class="MG17Motor" method="GetPosition_Position"(reference=w408, error in=w407, "lChanID"=w406) -> (reference out=w405:refnum<k7>, error out=w404:errorcluster, "GetPosition_Position"=w403:sgl)  [unwired: 1 in, 1 out]
        n163 = property on="Pos (mm)" class="DigNum (strict)"(error in=w402, "Value"=w401) -> (error out=w390:errorcluster)  [unwired: 1 in, 1 out]
        n164 = property on="Pos (mm)" class="DigNum (strict)"(error in=w397, "Value"=w396) -> (error out=w388:errorcluster)  [unwired: 1 in, 1 out]
        n165 = property on="Pos (mm)" class="DigNum (strict)"(error in=w404, "Value"=w403) -> (error out=w389:errorcluster)  [unwired: 1 in, 1 out]
        n166 = Bundle("Motor Reference"=w405, "Motor Reference"=w392, "Motor Reference"=w391) -> (w418:T14)  [unwired: 1 in]
        n167 = Merge Errors(w389, w390, w388) -> (w370:errorcluster)
        n168 = property on="InstrumentMode" class="Enum (strict)"("Value"=w371) -> ()  [unwired: 2 in, 2 out]
      }
      frame "BasicMode" {
        n169 = call-poly <vilib>:"Acquire Input Data.vi"("device ID"=w456, "Numeric"=w438, "error in (no error)"=w455) -> ("device ID 2"=w454:refnum<k1>, "axis info"=w450:T15, "button info"=w441:T16, "error out"=w439:errorcluster)  [unwired: 12 in, 1 out]
        n170 = call "j_GetJoystickSignal.vi"("RelJoyPos In"=w452, "NewJoystButtInfo"=w441, "NewJoystAxisInfo"=w450, "OldJoystButtInfo"=w440, "OldJoystickOffset"=w451) -> ("MoveZ"=→"Move Z":bool, "MoveXY"=→"Move XY":bool, "Joystick Offset"=w453:T3, "RelJoyPos"=w447:T4, "TalkToMotors?"=w444:bool)
        n171 = case shown="False" w444 {
          tunnel: w447 -> [w494 w498]
          tunnel: [w483 w515] -> w446
          tunnel: w445 -> [w493 w501]
          tunnel: w439 -> [w467 w500]
          tunnel: [w494 w498] -> w443
          frame False {
            # "Just Update Motor Position and Vel"
            n172 = Unbundle(w493) -> ("Motor Reference"=w492:refnum<k7>, "Motor Reference"=w485:refnum<k7>, "Motor Reference"=w484:refnum<k7>)
            n173 = property on="Pos (mm)" class="DigNum (strict)"(error in=w467) -> (error out=w475:errorcluster, "Value"=w472:sgl)  [unwired: 1 in, 1 out]
            n174 = property on="Pos (mm)" class="DigNum (strict)"(error in=w467) -> (error out=w468:errorcluster, "Value"=w465:sgl)  [unwired: 1 in, 1 out]
            n175 = property on="Pos (mm)" class="DigNum (strict)"(error in=w467) -> (error out=w476:errorcluster, "Value"=w481:sgl)  [unwired: 1 in, 1 out]
            n176 = invoke class="MG17Motor" method="GetPosition_Position"(reference=w485, error in=w475, "lChanID"=0) -> (error out=w488:errorcluster, "GetPosition_Position"=w473:sgl)  [unwired: 1 in, 2 out]
            n177 = invoke class="MG17Motor" method="GetPosition_Position"(reference=w484, error in=w468, "lChanID"=0) -> (error out=w486:errorcluster, "GetPosition_Position"=w464:sgl)  [unwired: 1 in, 2 out]
            n178 = property on="MotorLoopDelay" class="DigNum (strict)"() -> ("Value"=w460:u32)  [unwired: 2 in, 2 out]
            n179 = invoke class="MG17Motor" method="GetPosition_Position"(reference=w492, error in=w476, "lChanID"=0) -> (error out=w490:errorcluster, "GetPosition_Position"=w482:sgl)  [unwired: 1 in, 2 out]
            n180 = To Single Precision Float(number=w460) -> (single precision float=w459:sgl)
            n181 = Subtract(x=w482, y=w481) -> (x-y=w480:sgl)
            n182 = property on="Pos (mm)" class="DigNum (strict)"(error in=w488, "Value"=w473) -> (error out=w471:errorcluster)  [unwired: 1 in, 1 out]
            n183 = Subtract(x=w473, y=w472) -> (x-y=w474:sgl)
            n184 = Subtract(x=w464, y=w465) -> (x-y=w466:sgl)
            n185 = property on="Pos (mm)" class="DigNum (strict)"(error in=w486, "Value"=w464) -> (error out=w463:errorcluster)  [unwired: 1 in, 1 out]
            n186 = property on="Pos (mm)" class="DigNum (strict)"(error in=w490, "Value"=w482) -> (error out=w478:errorcluster)  [unwired: 1 in, 1 out]
            n187 = Divide(x=w459, y=sgl 1000.0) -> (x/y=w457:sgl)
            n188 = Divide(x=w480, y=w457) -> (x/y=w479:sgl)
            n189 = Divide(x=w474, y=w457) -> (x/y=w470:sgl)
            n190 = Divide(x=w466, y=w457) -> (x/y=w462:sgl)
            n191 = property on="Vel (mm/s)" class="DigNum (strict)"(error in=w478, "Value"=w479) -> (error out=w477:errorcluster)  [unwired: 1 in, 1 out]
            n192 = property on="Vel (mm/s)" class="DigNum (strict)"(error in=w471, "Value"=w470) -> (error out=w469:errorcluster)  [unwired: 1 in, 1 out]
            n193 = property on="Vel (mm/s)" class="DigNum (strict)"(error in=w463, "Value"=w462) -> (error out=w461:errorcluster)  [unwired: 1 in, 1 out]
            n194 = Merge Errors(w477, w469, w461) -> (w483:errorcluster)
          }
          frame True {
            # ">ZMotRef>"
            # ">YMotRef>"
            # ">XMotRef>"
            n195 = Unbundle By Name(w498) -> ("XRelPos"=w531:i32, "YRelPos"=w517:i32, "ZRelPos"=w502:i32)
            n196 = Unbundle(w501) -> ("Motor Reference"=w497:refnum<k7>, "Motor Reference"=w496:refnum<k7>, "Motor Reference"=w495:refnum<k7>)
            n197 = property on="Direction" class="DigNum (strict)"(error in=w500) -> (error out=w530:errorcluster, "Value"=w529:i32)  [unwired: 1 in, 1 out]
            n198 = property on="Direction" class="DigNum (strict)"(error in=w500) -> (error out=w520:errorcluster, "Value"=w519:i32)  [unwired: 1 in, 1 out]
            n199 = property on="Direction" class="DigNum (strict)"(error in=w500) -> (error out=w505:errorcluster, "Value"=w504:i32)  [unwired: 1 in, 1 out]
            n200 = property on="Move Z" class="Bool (strict)"(error in=w505) -> (error out=w513:errorcluster, "Value"=w512:bool)  [unwired: 1 in, 1 out]
            n201 = property on="Move XY" class="Bool (strict)"(error in=w530) -> (error out=w539:errorcluster, "Value"=w538:bool)  [unwired: 1 in, 1 out]
            n202 = property on="Move XY" class="Bool (strict)"(error in=w520) -> (error out=w528:errorcluster, "Value"=w527:bool)  [unwired: 1 in, 1 out]
            n203 = call "j_MotorExecute.vi"("MoveChamber?"=w538, "Axis Motor Settings"="X Motor Settings", "Error In"=w539, "JoystRelPos"=w531, "Motor's Old Direction"=w529, "Motor Reference In"=w497) -> ("Error Out"=w534:errorcluster, "Motor Position (mm)"=w533:sgl, "Motor's New Direction"=w532:i32, "Motor Velocity (mm/s)"=w535:sgl)  [unwired: 1 out]
            n204 = call "j_MotorExecute.vi"("MoveChamber?"=w527, "Axis Motor Settings"="Y Motor Settings", "Error In"=w528, "JoystRelPos"=w517, "Motor's Old Direction"=w519, "Motor Reference In"=w496) -> ("Error Out"=w523:errorcluster, "Motor Position (mm)"=w522:sgl, "Motor's New Direction"=w521:i32, "Motor Velocity (mm/s)"=w524:sgl)  [unwired: 1 out]
            n205 = call "j_MotorExecute.vi"("MoveChamber?"=w512, "Axis Motor Settings"="Z Motor Settings", "Error In"=w513, "JoystRelPos"=w502, "Motor's Old Direction"=w504, "Motor Reference In"=w495) -> ("Error Out"=w508:errorcluster, "Motor Position (mm)"=w507:sgl, "Motor's New Direction"=w506:i32, "Motor Velocity (mm/s)"=w509:sgl)  [unwired: 1 out]
            n206 = property on="Pos (mm)" class="DigNum (strict)"(error in=w534, "Value"=w533) -> (error out=w536:errorcluster)  [unwired: 1 in, 1 out]
            n207 = property on="Pos (mm)" class="DigNum (strict)"(error in=w523, "Value"=w522) -> (error out=w525:errorcluster)  [unwired: 1 in, 1 out]
            n208 = property on="Pos (mm)" class="DigNum (strict)"(error in=w508, "Value"=w507) -> (error out=w510:errorcluster)  [unwired: 1 in, 1 out]
            n209 = property on="Vel (mm/s)" class="DigNum (strict)"(error in=w536, "Value"=w535) -> (error out=w537:errorcluster)  [unwired: 1 in, 1 out]
            n210 = property on="Vel (mm/s)" class="DigNum (strict)"(error in=w525, "Value"=w524) -> (error out=w526:errorcluster)  [unwired: 1 in, 1 out]
            n211 = property on="Vel (mm/s)" class="DigNum (strict)"(error in=w510, "Value"=w509) -> (error out=w511:errorcluster)  [unwired: 1 in, 1 out]
            n212 = property on="Direction" class="DigNum (strict)"(error in=w526, "Value"=w521) -> (error out=w514:errorcluster)  [unwired: 1 in, 1 out]
            n213 = property on="Direction" class="DigNum (strict)"(error in=w537, "Value"=w532) -> (error out=w516:errorcluster)  [unwired: 1 in, 1 out]
            n214 = property on="Direction" class="DigNum (strict)"(error in=w511, "Value"=w506) -> (error out=w499:errorcluster)  [unwired: 1 in, 1 out]
            n215 = Merge Errors(w516, w514, w499) -> (w515:errorcluster)
          }
        }
        n216 = property on="InstrumentMode" class="Enum (strict)"() -> ("Value"=w442:T2)  [unwired: 2 in, 2 out]
      }
      frame "PassiveMode" {
        n217 = property on="InstrumentMode" class="Enum (strict)"() -> ("Value"=w547:T2)  [unwired: 2 in, 2 out]
      }
      frame "AcquireOffsetMode" {
        n218 = property on="InstrumentMode" class="Enum (strict)"() -> ("Value"=w554:T2)  [unwired: 2 in, 2 out]
      }
      frame "AcquireSpectrumMode" {
        n219 = property on="InstrumentMode" class="Enum (strict)"() -> ("Value"=w561:T2)  [unwired: 2 in, 2 out]
      }
      frame "Force-ExtensionMode" {
        n220 = property on="InstrumentMode" class="Enum (strict)"() -> ("Value"=w568:T2)  [unwired: 2 in, 2 out]
      }
      frame "Shutdown" {
        n221 = call-poly <vilib>:"Close Input Device.vi"("error in (no error)"=w572, "device ID"=w571) -> ("error out"=w580:errorcluster)  [unwired: 8 in]
        n222 = Unbundle(w573) -> ("Motor Reference"=w576:refnum<k7>, "Motor Reference"=w575:refnum<k7>, "Motor Reference"=w574:refnum<k7>)
        n223 = call "s_CloseMotor.vi"("Error In"=w580, "Motor Reference In"=w576) -> ("Error Out"=w585:errorcluster)
        n224 = call "s_CloseMotor.vi"("Error In"=w580, "Motor Reference In"=w575) -> ("Error Out"=w583:errorcluster)
        n225 = call "s_CloseMotor.vi"("Error In"=w580, "Motor Reference In"=w574) -> ("Error Out"=w581:errorcluster)
        n226 = property on="IsActive?" class="Bool (strict)"(error in=w585, "Value"=FALSE ("IsYMotorActive?")) -> (error out=w579:errorcluster)  [unwired: 1 in, 1 out]
        n227 = property on="IsActive?" class="Bool (strict)"(error in=w583, "Value"=FALSE ("IsYMotorActive?")) -> (error out=w578:errorcluster)  [unwired: 1 in, 1 out]
        n228 = property on="IsActive?" class="Bool (strict)"(error in=w581, "Value"=FALSE ("IsYMotorActive?")) -> (error out=w577:errorcluster)  [unwired: 1 in, 1 out]
        n229 = Merge Errors(w579, w578, w577) -> (w570:errorcluster)
        n230 = property on="InstrumentMode" class="Enum (strict)"(error in=w570) -> (error out=w569:errorcluster, "Value"=w587:T2)  [unwired: 1 in, 1 out]
      }
    }
    n231 = Wait (ms)(milliseconds to wait=u32 2000) -> ()  [unwired: 1 out]
  }
